vi "single-axis scan settings.vi"(8 "Error In":errorcluster, 10 "General information in":T2 {"axis to scan" items=["X", "Y", "Z"]; "channel for fit" min=0 max=20; "scan end position" min=0.0 max=105.0; "scan start position" min=0.0 max=105.0}, 11 "Action (R)":T1=enum."read") -> (0 "Error out":errorcluster, 2 "general information out":T2 {"axis to scan" items=["X", "Y", "Z"]; "channel for fit" min=0 max=20; "scan end position" min=0.0 max=105.0; "scan start position" min=0.0 max=105.0})   [LabVIEW 2011]
doc: "Functional Global Variable for the algorithm settings. The used method as well as the max. Iteration steps and the tolerance can be given. In addition, the algorithm can be told to use boundaries (if possible)."
uses:
  controls/x-scan settings.ctl
  controls/FGV_Action.ctl
panel:
  # "Input"
  # "Output"
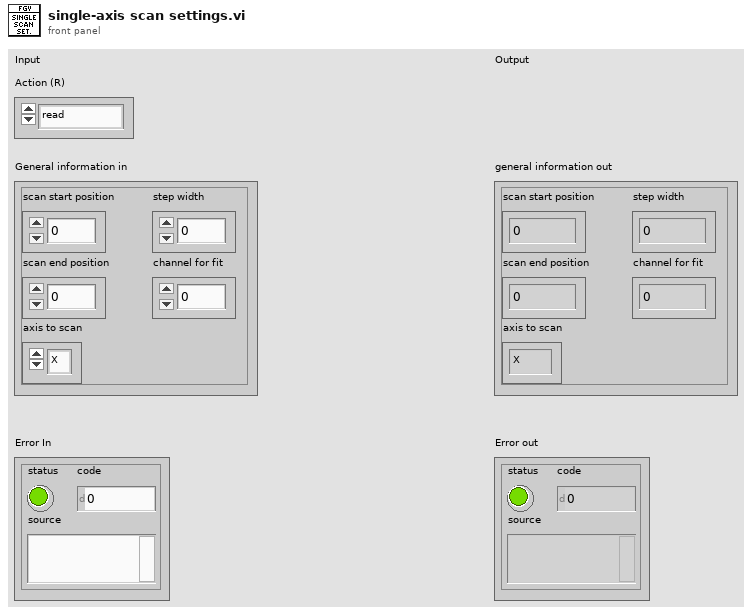
[diagram p1: front panel]
types:
  T1 = typedef "FGV_Action.ctl" = enum16{"set to default", "read", "write"}
  T2 = typedef "x-scan settings.ctl" = cluster{"scan start position":dbl, "scan end position":dbl, "step width":dbl, "channel for fit":i32, "axis to scan":u16}
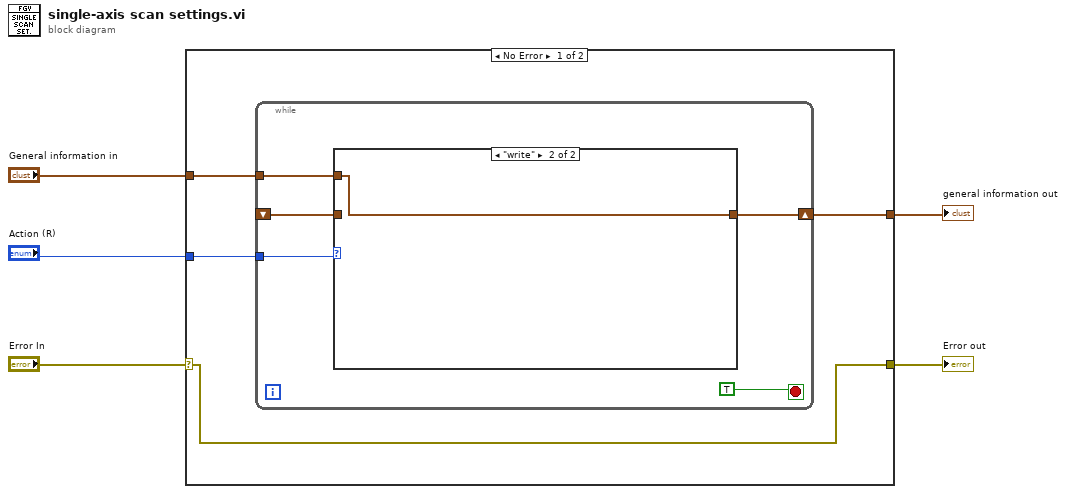
[diagram p0: block diagram]
diagram:
  n1 = case shown="No Error" "Error In" {
    selector: "Error In" -> [w6 w18]
    tunnel: "Action (R)" -> [w9 _]
    tunnel: [w6 w18] -> w4
    tunnel: "General information in" -> [w8 w17]
    tunnel: [w7 w17] -> w2
    frame No Error {
      n2 = while {
        tunnel: w9 -> [w13]
        tunnel: w8 -> [w12]
        shift-right: [w10] -> w7
        shift-left: _ -> [w11]
        stop <- TRUE stop-if-true
        n3 = case shown="\"write\"" w13 {
          tunnel: w12 -> [_ w16]
          tunnel: w11 -> [w15 _]
          tunnel: [w15 w16] -> w10
          frame "read", Default {
          }
          frame "write" {
          }
        }
      }
    }
    frame Error {
    }
  }
  "Error out" <- w4
  "general information out" <- w2
